vi "BRig_dataAnalog_iState_start.vi"() -> (2 "output_iState_start":i32)   [LabVIEW 2014]
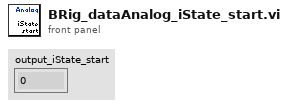
[diagram p1: front panel]
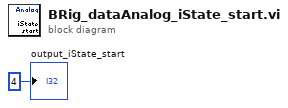
[diagram p0: block diagram]
diagram:
  "output_iState_start" <- 4 ("output_iBlock")
